vi "Test Result Properties.vi"(11 "NI SystemLink Test Result in":refnum<class "NI SystemLink Test Result.lvclass">) -> (3 "Array":T1[](array[typedef]))   [LabVIEW 2023, in "Logger.lvclass"]
uses:
  Logger.lvclass
  <vilib>/Skyline/Tag/Shared/typedefs/TagProperty.ctl
  <vilib>/Skyline/TestMonitor/Test Result/NI SystemLink Test Result.lvclass
  <vilib>/Skyline/TestMonitor/Test Result/NI SystemLink Test Result.lvclass/NI SystemLink Test Result.ctl
  <vilib>/Skyline/TestMonitor/Test Result/Read Part Number.vi
  <vilib>/Skyline/TestMonitor/Test Result/Read Serial Number.vi
  <vilib>/Skyline/TestMonitor/Test Result/Read Operator.vi
  <vilib>/Skyline/TestMonitor/Test Result/Read Id.vi
  <vilib>/Skyline/TestMonitor/Test Result/Read Host Name.vi
  <vilib>/Skyline/TestMonitor/Test Result/Read Program Name.vi
  <vilib>/Skyline/Tag/Shared/NI Skyline Tag.lvlib
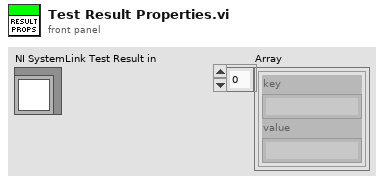
[diagram p1: front panel]
types:
  T1 = typedef "NI Skyline Tag.lvlib/TagProperty.ctl" = cluster{"key":string, "value":string}
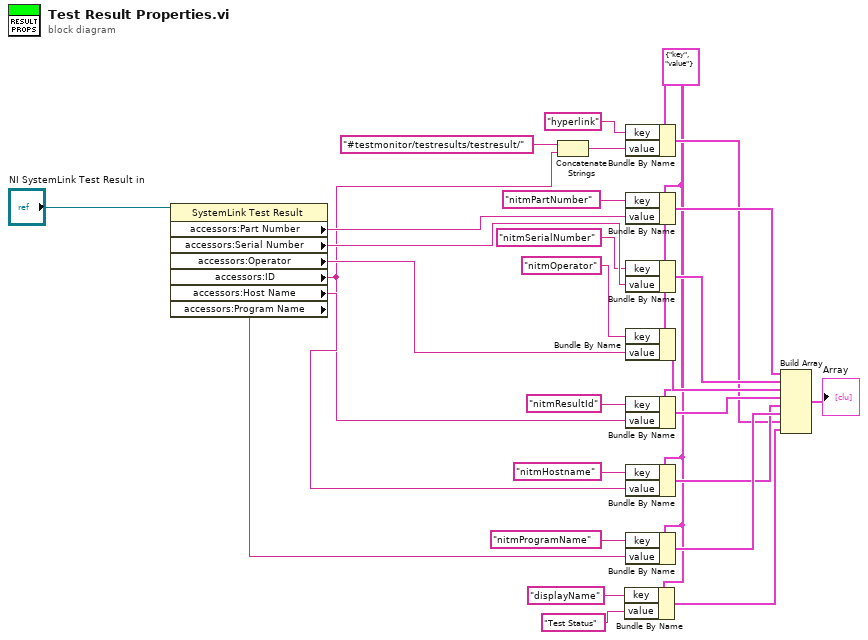
[diagram p0: block diagram]
diagram:
  w4 = T1 {"key"="key", "value"="value"} ("Property")
  n1 = property class="SystemLink Test Result"(reference="NI SystemLink Test Result in") -> ("accessors:Part Number"=w13:string, "accessors:Serial Number"=w15:string, "accessors:Operator"=w25:string, "accessors:ID"=w7:string, "accessors:Host Name"=w26:string, "accessors:Program Name"=w27:string)  [unwired: 1 in, 2 out]
  n2 = Concatenate Strings("#testmonitor/testresults/testresult/" ("key"), w7) -> (w6:string)
  n3 = Bundle By Name(cluster=w4, "key"="displayName", "value"="Test Status") -> (w3:T1)
  n4 = Bundle By Name(cluster=w4, "key"="hyperlink", "value"=w6) -> (w5:T1)
  n5 = Bundle By Name(cluster=w4, "key"="nitmPartNumber", "value"=w13) -> (w11:T1)
  n6 = Bundle By Name(cluster=w4, "key"="nitmSerialNumber", "value"=w15) -> (w20:T1)
  n7 = Bundle By Name(cluster=w4, "key"="nitmOperator", "value"=w25) -> (w21:T1)
  n8 = Bundle By Name(cluster=w4, "key"="nitmResultId", "value"=w7) -> (w22:T1)
  n9 = Bundle By Name(cluster=w4, "key"="nitmHostname", "value"=w26) -> (w23:T1)
  n10 = Bundle By Name(cluster=w4, "key"="nitmProgramName", "value"=w27) -> (w24:T1)
  n11 = Build Array(w11, w20, w21, w22, w23, w24, w5, w3) -> (→"Array":T1[])
